vi "CRYPEAQ adapt.vi"(0 "EhsR":dbl[](array[numeric]), 1 "fc":dbl[](array[numeric]), 3 "Nc":i32, 5 "EhsT":dbl[](array[numeric]), 7 "Model":u16(ring) items=["FFT", "Other"], 9 "Version":u16(ring) items=["Basic", "Advance", "Default"], 12 "Fs":dbl=2048.0, 14 "NF":dbl=2048.0) -> (4 "EpR":dbl[](array[numeric]), 6 "EpT":dbl[](array[numeric]))   [LabVIEW 2013]
uses:
  CRYPEAQ Global.vi
panel:
  out "Adapted Signal":cluster{dbl[], "EpR":dbl[]}[](graph)
  out "Origin Signal":cluster{dbl[], "EpR":dbl[]}[](graph)
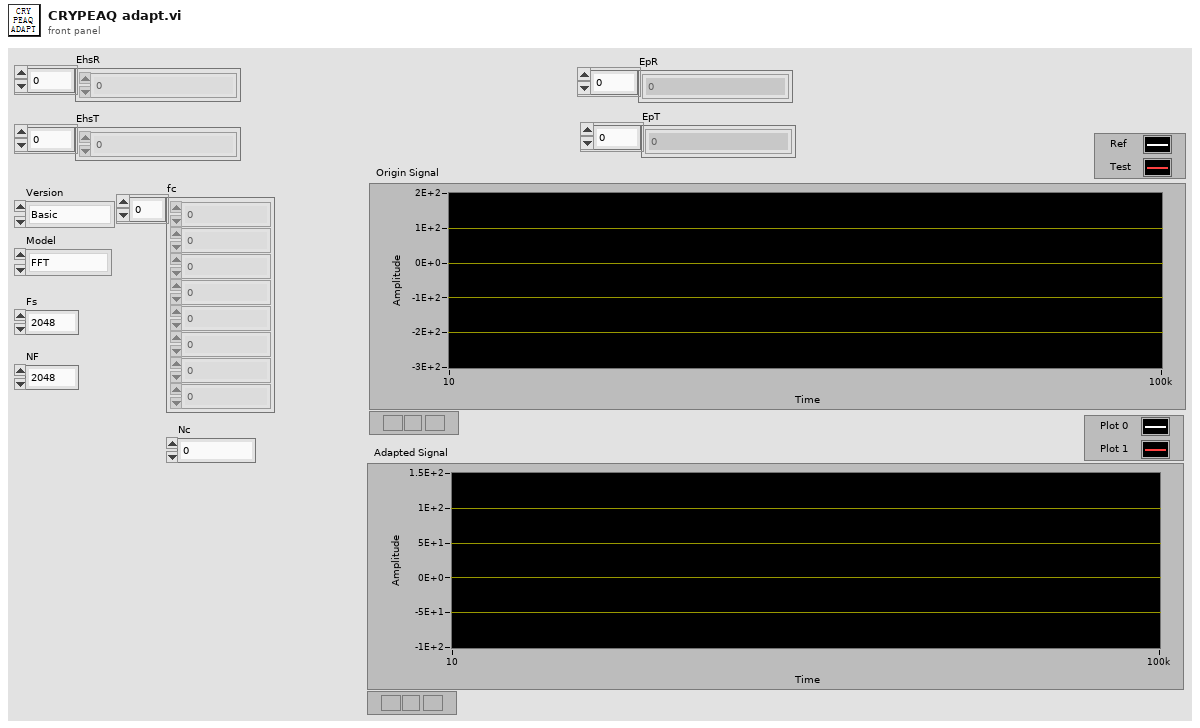
[diagram p1: front panel]
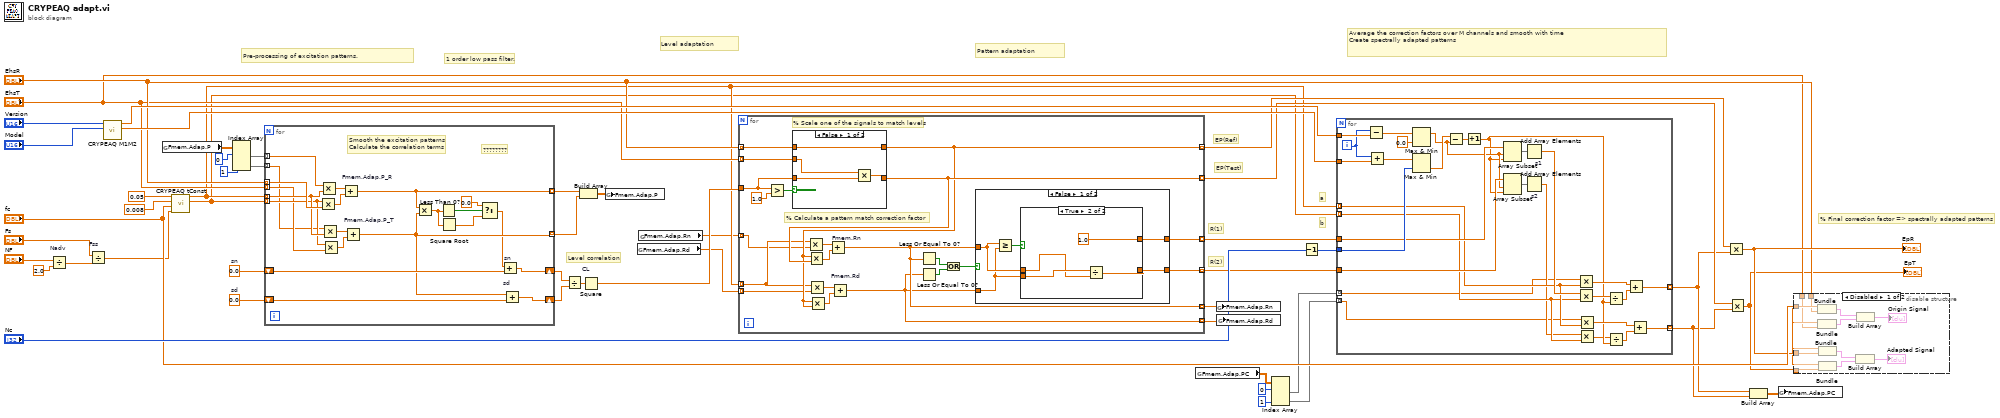
[diagram p0: block diagram]
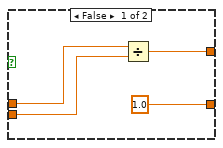
[diagram p3: hidden frame]
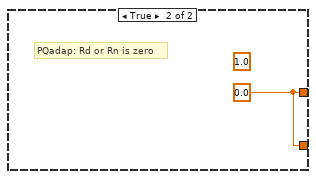
[diagram p4: hidden frame]
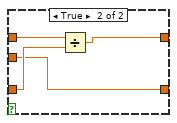
[diagram p5: hidden frame]
diagram:
  w43 = 0.0  # sd
  w44 = 0.0  # sn
  # "Average the correction factors over M channels and smooth with time\nCreate spectrally adapted patterns"
  # "% Final correction factor => spectrally adapted patterns"
  # "b"
  # "a"
  # "R(2)"
  # "R(1)"
  # "1 order low pass filter."
  # "EP(Test)"
  # "EP(Ref)"
  # "Pattern adaptation"
  # "Level adaptation"
  # "Pre-processing of excitation patterns."
  # "Level correlation"
  n1 = Divide "Nadv"(x="NF", y=2.0) -> (x/y=w46:dbl)
  n2 = Divide "Fss"(x="Fs", y=w46) -> (x/y=w22:dbl)
  n3 = call "CRYPEAQ M1M2.vi"("Model"="Model", "Version"="Version") -> ("M2"=w37:dbl, "M1"=w38:dbl)  [unwired: 8 in]
  n4 = global read "CRYPEAQ Global.vi" "Fmem.Adap.P"() -> (w21:dbl[][])
  n5 = call "CRYPEAQ tConst.vi"("Fss"=w22, "f(fc)"="fc", "tmin"=0.008, "t100"=0.05) -> ("b"=w1:dbl[], "a"=w24:dbl[])  [unwired: 6 in]
  n6 = Index Array(array=w21, index (row) #1=0 ("index (row)"), index (row) #2=1 ("index (row)")) -> (element #1=w4:dbl[], element #2=w18:dbl[])  [unwired: 2 in]
  n7 = for {
    tunnel: "EhsR" -> [w70] mode=indexing
    tunnel: "EhsT" -> [w64] mode=indexing
    tunnel: w24 -> [w66] mode=indexing
    tunnel: w1 -> [w65] mode=indexing
    shift-right: [w60] -> w42
    shift-left: w44 -> [w63]
    shift-right: [w61] -> w41
    shift-left: w43 -> [w62]
    tunnel: w4 -> [w57] mode=indexing
    tunnel: w18 -> [w56] mode=indexing
    tunnel: [w55] -> w17 mode=indexing
    tunnel: [w54] -> w16 mode=indexing
    # "????????"
    # "Smooth the excitation patterns\nCalculate the correlation terms"
    n8 = Multiply(x=w65, y=w70) -> (x*y=w69:dbl)
    n9 = Multiply(x=w57, y=w66) -> (x*y=w71:dbl)
    n10 = Multiply(x=w56, y=w66) -> (x*y=w67:dbl)
    n11 = Multiply(x=w65, y=w64) -> (x*y=w68:dbl)
    n12 = Add "Fmem.Adap.P_R"(x=w71, y=w69) -> (x+y=w55:dbl)
    n13 = Add "Fmem.Adap.P_T"(x=w67, y=w68) -> (x+y=w54:dbl)
    n14 = Multiply(x=w55, y=w54) -> (x*y=w58:dbl)
    n15 = Less Than 0?(x=w58) -> (x < 0?=w59:bool)
    n16 = Square Root(x=w58) -> (sqrt(x)=w53:dbl)
    n17 = Select(t=0.0, s=w59, f=w53) -> (s? t:f=w52:dbl)
    n18 = Add "sn"(x=w52, y=w63) -> (x+y=w60:dbl)
    n19 = Add "sd"(x=w54, y=w62) -> (x+y=w61:dbl)
  }
  n20 = Divide(x=w42, y=w41) -> (x/y=w40:dbl)
  n21 = Build Array(w17, w16) -> (w15:dbl[][])
  n22 = Square "CL"(x=w40) -> (x^2=w39:dbl)
  n23 = global write "CRYPEAQ Global.vi" "Fmem.Adap.P"(w15) -> ()
  n24 = global read "CRYPEAQ Global.vi" "Fmem.Adap.Rd"() -> (w3:dbl[])
  n25 = global read "CRYPEAQ Global.vi" "Fmem.Adap.Rn"() -> (w14:dbl[])
  n26 = for {
    tunnel: w39 -> [w90]
    tunnel: "EhsR" -> [w86] mode=indexing
    tunnel: "EhsT" -> [w85] mode=indexing
    tunnel: [w82] -> w29 mode=indexing
    tunnel: [w83] -> w25 mode=indexing
    tunnel: w24 -> [w81] mode=indexing
    tunnel: [w80] -> w23 mode=indexing
    tunnel: [w79] -> w35 mode=indexing
    tunnel: w14 -> [w75] mode=indexing
    tunnel: w3 -> [w74] mode=indexing
    tunnel: [w73] -> w13 mode=indexing
    tunnel: [w72] -> w12 mode=indexing
    # "% Calculate a pattern match correction factor"
    # "% Scale one of the signals to match levels"
    n27 = Greater?(x=w90, y=1.0) -> (0:w91:bool)
    n28 = case shown="False" w91 {
      tunnel: w90 -> [w108 w112]
      tunnel: w86 -> [w110 w114]
      tunnel: [w110 w113] -> w82
      tunnel: w85 -> [w109 w111]
      tunnel: [w107 w111] -> w83
      frame False {
        n29 = Multiply(x=w109, y=w108) -> (x*y=w107:dbl)
      }
      frame True {
        n30 = Divide(x=w114, y=w112) -> (x/y=w113:dbl)
      }
    }
    n31 = Multiply(x=w81, y=w75) -> (x*y=w87:dbl)
    n32 = Multiply(x=w82, y=w83) -> (x*y=w84:dbl)
    n33 = Multiply(x=w81, y=w74) -> (x*y=w89:dbl)
    n34 = Multiply(x=w82, y=w82) -> (x*y=w88:dbl)
    n35 = Add "Fmem.Rn"(x=w87, y=w84) -> (x+y=w73:dbl)
    n36 = Add "Fmem.Rd"(x=w89, y=w88) -> (x+y=w72:dbl)
    n37 = Less Or Equal To 0?(x=w73) -> (x <= 0?=w78:bool)
    n38 = Less Or Equal To 0?(x=w72) -> (x <= 0?=w77:bool)
    n39 = Or(x=w78, y=w77) -> (x .or. y?=w76:bool)
    n40 = case shown="False" w76 {
      tunnel: [w96 w106] -> w80
      tunnel: [w95 w106] -> w79
      tunnel: w73 -> [w94 _]
      tunnel: w72 -> [w93 _]
      frame False {
        n41 = Greater Or Equal?(x=w94, y=w93) -> (x >= y?=w97:bool)
        n42 = case shown="True" w97 {
          tunnel: [1.0 ("x+y") w104] -> w96
          tunnel: [w98 1.0 ("x+y")] -> w95
          tunnel: w94 -> [w100 w102]
          tunnel: w93 -> [w99 w103]
          frame False {
            n43 = Divide(x=w100, y=w99) -> (x/y=w98:dbl)
          }
          frame True {
            n44 = Divide(x=w103, y=w102) -> (x/y=w104:dbl)
          }
        }
      }
      frame True {
        (unwired) 1.0 ("x+y")
        w106 = 0.0 ("x+y")
        # "PQadap: Rd or Rn is zero"
      }
    }
  }
  n45 = global read "CRYPEAQ Global.vi" "Fmem.Adap.PC"() -> (w11:dbl[][])
  n46 = global write "CRYPEAQ Global.vi" "Fmem.Adap.Rn"(w13) -> ()
  n47 = global write "CRYPEAQ Global.vi" "Fmem.Adap.Rd"(w12) -> ()
  n48 = Index Array(array=w11, index (row) #1=0 ("index (row)"), index (row) #2=1 ("index (row)")) -> (element #1=w8:dbl[], element #2=w2:dbl[])  [unwired: 2 in]
  n49 = Decrement(x="Nc") -> (x-1=w36:i32)
  n50 = for {
    tunnel: w38 -> [w143]
    tunnel: w37 -> [w141]
    tunnel: w36 -> [w137]
    tunnel: w35 -> [w133]
    tunnel: w23 -> [w131]
    tunnel: w24 -> [w125] mode=indexing
    tunnel: w1 -> [w118] mode=indexing
    tunnel: [w124] -> w6 mode=indexing
    tunnel: [w123] -> w5 mode=indexing
    tunnel: w8 -> [w115] mode=indexing
    tunnel: w2 -> [w116] mode=indexing
    i -> [w142]
    n51 = Subtract(x=w142, y=w143) -> (x-y=w139:dbl)
    n52 = Add(x=w142, y=w141) -> (x+y=w140:dbl)
    n53 = Max & Min(x=w140, y=w137) -> (min(x,y)=w136:dbl)  [unwired: 1 out]
    n54 = Max & Min(x=w139, y=0.0) -> (max(x,y)=w130:dbl)  [unwired: 1 out]
    n55 = Subtract(x=w136, y=w130) -> (x-y=w135:dbl)
    n56 = Increment(x=w135) -> (x+1=w120:dbl)
    n57 = Array Subset(array=w133, index=w130, length=w120) -> (w134:dbl[])
    n58 = Array Subset(array=w131, index=w130, length=w120) -> (w132:dbl[])
    n59 = Add Array Elements "s1"(numeric array=w134) -> (sum=w129:dbl)
    n60 = Add Array Elements "s2"(numeric array=w132) -> (sum=w117:dbl)
    n61 = Multiply(x=w115, y=w125) -> (x*y=w126:dbl)
    n62 = Multiply(x=w129, y=w118) -> (x*y=w128:dbl)
    n63 = Multiply(x=w116, y=w125) -> (x*y=w122:dbl)
    n64 = Multiply(x=w117, y=w118) -> (x*y=w119:dbl)
    n65 = Divide(x=w128, y=w120) -> (x/y=w127:dbl)
    n66 = Divide(x=w119, y=w120) -> (x/y=w121:dbl)
    n67 = Add(x=w126, y=w127) -> (x+y=w124:dbl)
    n68 = Add(x=w122, y=w121) -> (x+y=w123:dbl)
  }
  n69 = Multiply(x=w29, y=w6) -> (x*y=w31:dbl[])
  "EpR" <- w31
  n70 = Multiply(x=w25, y=w5) -> (x*y=w26:dbl[])
  "EpT" <- w26
  n71 = Build Array(w6, w5) -> (w7:dbl[][])
  n72 = global write "CRYPEAQ Global.vi" "Fmem.Adap.PC"(w7) -> ()
  n73 = disable-structure shown="Disabled" {
    disable-tunnel: "fc" -> [w148 _]
    disable-tunnel: w31 -> [w147 _]
    disable-tunnel: "EhsR" -> [w146 _]
    disable-tunnel: "EhsT" -> [w145 _]
    disable-tunnel: w26 -> [w144 _]
    frame Disabled {
      n74 = Bundle("fc"=w148, "EhsR"=w146) -> (w154:cluster{"fc":dbl[], "EhsR":dbl[]})  [unwired: 1 in]
      n75 = Bundle("fc"=w148, "EhsT"=w145) -> (w153:cluster{"fc":dbl[], "EhsT":dbl[]})  [unwired: 1 in]
      n76 = Bundle("fc"=w148, w147) -> (w149:cluster{"fc":dbl[], dbl[]})  [unwired: 1 in]
      n77 = Bundle("fc"=w148, w144) -> (w150:cluster{"fc":dbl[], dbl[]})  [unwired: 1 in]
      n78 = Build Array(w149, w150) -> (→"Adapted Signal":cluster{"fc":dbl[], dbl[]}[])
      n79 = Build Array(w154, w153) -> (→"Origin Signal":cluster{"fc":dbl[], "EhsT":dbl[]}[])
    }
    frame Enabled {
    }
  }
